vi "快捷创建.C.H文件.vi"() -> ()   [LabVIEW 2019]
panel:
  in  "取消按钮":bool
  in  "新建按钮":bool
  in  "输入文件名":string
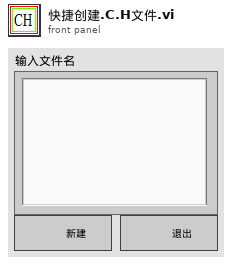
[diagram p1: front panel]
types:
  T1 = enum16{"open", "replace", "create", "open or create", "replace or create", "replace or create with confirmation"}
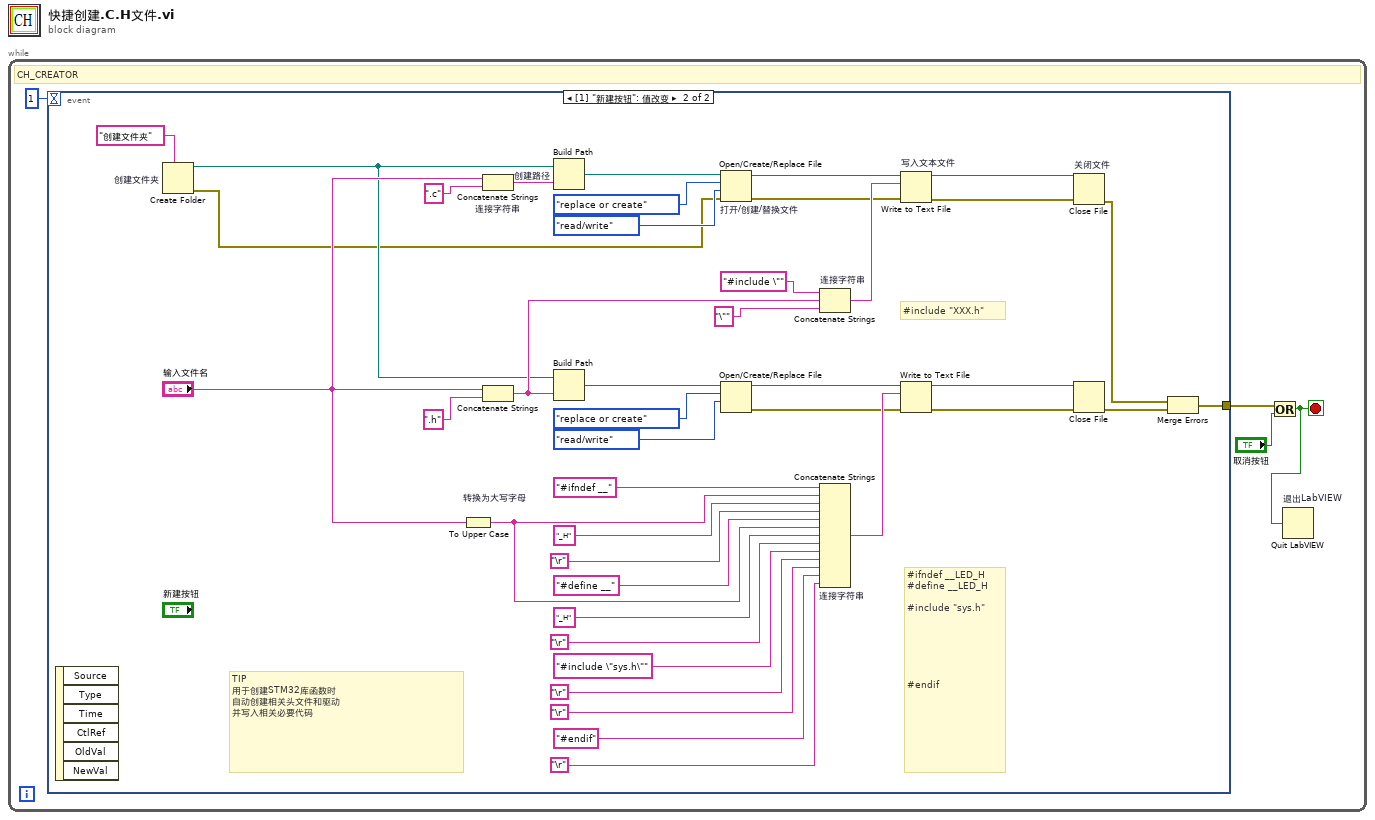
[diagram p0: block diagram]
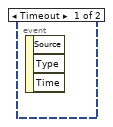
[diagram p2: hidden frame]
diagram:
  n1 = while {
    stop <- w1 stop-if-true
    # "CH_CREATOR"
    n2 = event shown="[1] \"新建按钮\": 值改变" {
      selector: _ -> [_ _]
      dyn-events: _ -> [_ _]
      timeout: 1 -> [_ _]
      tunnel: [_ w5] -> w3
      event Timeout {
        n3 = event-data() -> ()  [unwired: 1 in, 3 out]
      }
      event "新建按钮": Value Change {
        # "TIP\n用于创建STM32库函数时\n自动创建相关头文件和驱动\n并写入相关必要代码"
        # "#include \"XXX.h\""
        # "#ifndef __LED_H\n#define __LED_H\n\n#include \"sys.h\"\n\n\n\n\n\n\n#endif"
        n4 = event-data() -> ()  [unwired: 1 in, 6 out]
        n5 = Create Folder "创建文件夹"(prompt (Create Folder)="创建文件夹" ("对话框窗口（创建文件夹）")) -> (created path=w12:path, error out=w8:errorcluster)  [unwired: 2 in, 1 out]
        n6 = To Upper Case "转换为大写字母"(1:"输入文件名") -> (0:w41:string)
        n7 = Concatenate Strings "连接字符串"("输入文件名", ".c" ("字符串")) -> (w32:string)
        n8 = Concatenate Strings("输入文件名", ".h" ("字符串")) -> (w36:string)
        n9 = Build Path "创建路径"(base path=w12, name or relative path=w32) -> (appended path=w33:path)
        n10 = Build Path(base path=w12, name or relative path=w36) -> (appended path=w34:path)
        n11 = Open/Create/Replace File "打开/创建/替换文件"(file path (use dialog)=w33, error in=w8, operation (0:open)=T1."replace or create" ("操作(0:open)"), access (0:read/write)=enum16{"read/write", "read-only", "write-only"}."read/write" ("权限(0:read/write)")) -> (refnum out=w35:refnum<file>, error out=w9:errorcluster)  [unwired: 2 in, 1 out]
        n12 = Open/Create/Replace File(file path (use dialog)=w34, operation (0:open)=T1."replace or create" ("操作(0:open)"), access (0:read/write)=enum16{"read/write", "read-only", "write-only"}."read/write" ("权限(0:read/write)")) -> (refnum out=w38:refnum<file>, error out=w10:errorcluster)  [unwired: 3 in, 1 out]
        n13 = Concatenate Strings "连接字符串"("#include \"" ("字符串"), w36, "\"" ("字符串")) -> (w37:string)
        n14 = Concatenate Strings "连接字符串"("#ifndef __" ("字符串"), w41, "_H" ("字符串"), "\r", "#define __" ("字符串"), w41, "_H" ("字符串"), "\r", "#include \"sys.h\"" ("字符串"), "\r", "\r", "#endif" ("字符串"), "\r") -> (w39:string)
        n15 = Write to Text File "写入文本文件"(file (use dialog)=w35, text=w37, error in=w9) -> (refnum out=w42:refnum<file>, error out=w43:errorcluster)  [unwired: 1 in, 1 out]
        n16 = Write to Text File(file (use dialog)=w38, text=w39, error in=w10) -> (refnum out=w44:refnum<file>, error out=w45:errorcluster)  [unwired: 1 in, 1 out]
        n17 = Close File "关闭文件"(refnum=w42, error in=w43) -> (error out=w7:errorcluster)  [unwired: 1 out]
        n18 = Close File(refnum=w44, error in=w45) -> (error out=w6:errorcluster)  [unwired: 1 out]
        n19 = Merge Errors(w7, w6) -> (w5:errorcluster)
      }
    }
    n20 = Or(x=w3, y="取消按钮") -> (x .or. y?=w1:bool)
    n21 = Quit LabVIEW "退出LabVIEW"(quit? (T)=w1) -> ()
  }
